vi "Check Aircraft UDP Port.vi"(8 "Error In":errorcluster, 11 "Aircraft ID":u8) -> (0 "Error Out":errorcluster, 3 "Downlink Port Found":bool)   [LabVIEW 2014]
uses:
  Get Aircraft Information.vi
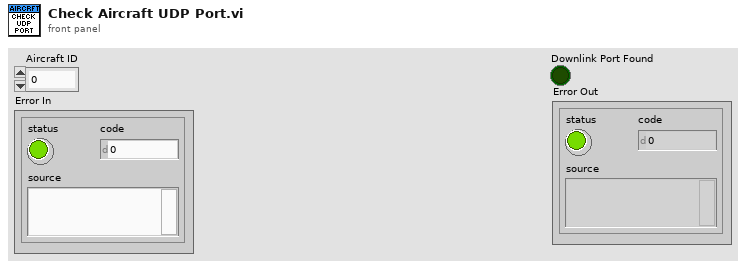
[diagram p1: front panel]
types:
  T1 = typedef "Drone Information.ctl" = cluster{"Heart Beat":bool, "Aircraft ID":u8, "Downlink Port":refnum<visa-resource-name>, "Tag ID":string, "System Status":string, "Base Mode":T2, "Armed/Disarmed":bool, "Battery Voltage":dbl, "Control Mode":T3, "Initialisation":u8, "Heart Beat Status":bool, "Uplink Port":refnum<visa-resource-name>, "UDP connection ID":refnum<k16>, "Connection Type":T4, "Mode":string, "UDP IP Address":string, "Mission Uploaded":bool}
  T2 = typedef "Base Mode.ctl" = cluster{"Custom Mode":bool, "Test Enabled":bool, "Autonomous Mode":bool, "Guided Mode":bool, "Stabilization Enabled":bool, "HIL Enabled":bool, "Manual Mode":bool, "Arm":bool}
  T3 = typedef "Aircraft Mode.ctl" = enum16{"Loiter", "Stabalise", "Failsafe", "Emergency Stop"}
  T4 = typedef "Telemetry Connection Type.ctl" = enum16{"Serial", "UDP", "TCP"}
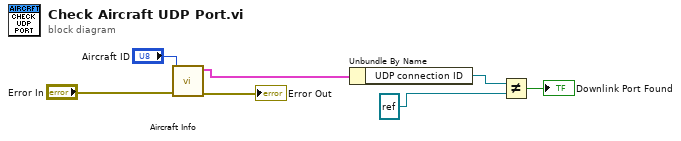
[diagram p0: block diagram]
diagram:
  n1 = call-poly "Aircraft Info.vi"("Error In"="Error In", "Aircraft ID"="Aircraft ID") -> ("Error Out"=→"Error Out":errorcluster, "Aircraft Information Out"=w6:T1)  [unwired: 8 in]
  n2 = Unbundle By Name(w6) -> ("UDP connection ID"=w5:refnum<k16>)
  n3 = Not Equal?(x=w5, y=refnum<k16> refnum) -> (x != y?=→"Downlink Port Found":bool)
